vi "Example0.vi"() -> ()   [LabVIEW 2016]
panel:
  in  "Numeric 2":dbl
  in  "Dial":dbl(knob) scale=0.0..10.0
  in  "Numeric":dbl
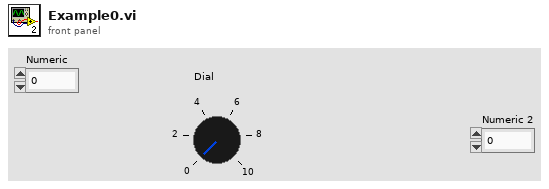
[diagram p1: front panel]
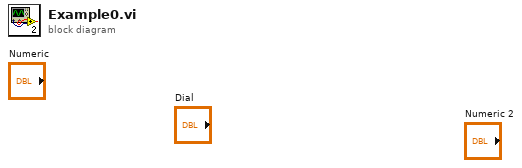
[diagram p0: block diagram]
diagram:
